vi "输入输出力计算.vi"(6 "测量点数组":dbl[](array[numeric]), 7 "滞后监控点":dbl, 8 "左下降数组":dbl[][](array[numeric]), 9 "左上升数组":dbl[][](array[numeric]), 10 "右下降数组":dbl[][](array[numeric]), 11 "右上升数组":dbl[][](array[numeric])) -> (1 "扭差":dbl, 2 "左扭矩数组":dbl[](array[numeric]), 3 "右扭矩数组":dbl[](array[numeric]), 4 "左滞后":dbl, 5 "右滞后":dbl)   [LabVIEW 2011]
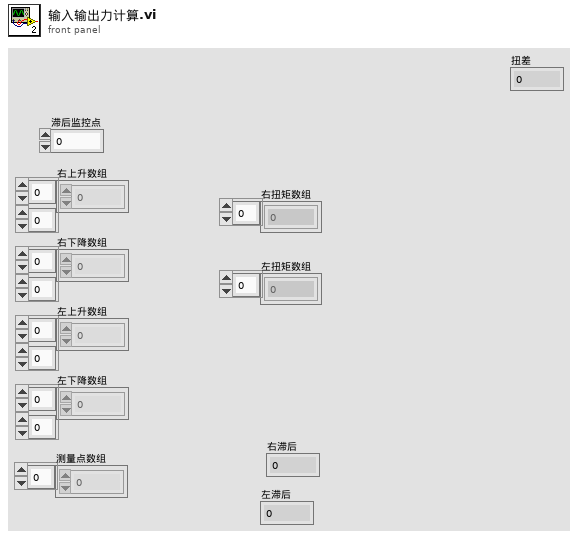
[diagram p1: front panel]
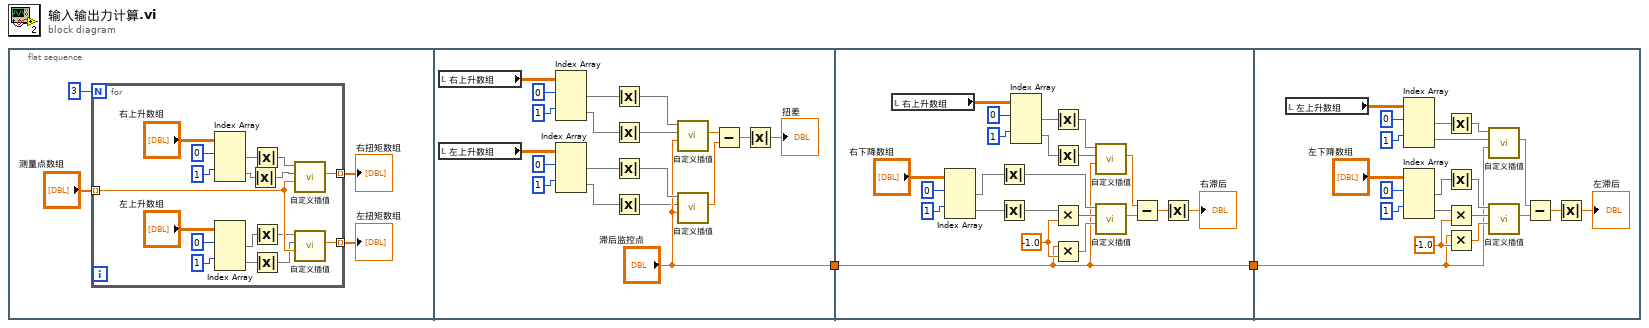
[diagram p0: block diagram]
diagram:
  n1 = flat-sequence {
    tunnel: ["滞后监控点"] -> w1
    tunnel: [w47] -> w2
    tunnel: w1 -> [w47]
    tunnel: w2 -> [w67]
    frame #0 {
      n2 = for {
        N: 3 -> [_]
        tunnel: "测量点数组" -> [w19] mode=indexing
        tunnel: [w14] -> w4 mode=indexing
        tunnel: [w13] -> w3 mode=indexing
        n3 = Index Array(array="右上升数组", index (row) #1=0 ("索引 (行)"), index (row) #2=1 ("索引 (行)")) -> (element #1=w18:dbl[], element #2=w8:dbl[])  [unwired: 2 in]
        n4 = Index Array(array="左上升数组", index (row) #1=0 ("索引 (行)"), index (row) #2=1 ("索引 (行)")) -> (element #1=w16:dbl[], element #2=w10:dbl[])  [unwired: 2 in]
        n5 = Absolute Value(x=w8) -> (abs(x)=w7:dbl[])
        n6 = Absolute Value(x=w18) -> (abs(x)=w17:dbl[])
        n7 = Absolute Value(x=w16) -> (abs(x)=w15:dbl[])
        n8 = Absolute Value(x=w10) -> (abs(x)=w9:dbl[])
        n9 = call "自定义插值.vi"("压力"=w19, "压力数组"=w7, "扭矩数组"=w17) -> ("扭矩值"=w14:dbl)  [unwired: 8 in]
        n10 = call "自定义插值.vi"("压力"=w19, "压力数组"=w9, "扭矩数组"=w15) -> ("扭矩值"=w13:dbl)  [unwired: 8 in]
      }
      "右扭矩数组" <- w4
      "左扭矩数组" <- w3
    }
    frame #1 {
      n11 = local read "右上升数组"() -> (w40:dbl[][])
      n12 = local read "左上升数组"() -> (w37:dbl[][])
      n13 = Index Array(array=w40, index (row) #1=0 ("索引 (行)"), index (row) #2=1 ("索引 (行)")) -> (element #1=w36:dbl[], element #2=w25:dbl[])  [unwired: 2 in]
      n14 = Index Array(array=w37, index (row) #1=0 ("索引 (行)"), index (row) #2=1 ("索引 (行)")) -> (element #1=w33:dbl[], element #2=w27:dbl[])  [unwired: 2 in]
      n15 = Absolute Value(x=w36) -> (abs(x)=w35:dbl[])
      n16 = Absolute Value(x=w25) -> (abs(x)=w24:dbl[])
      n17 = Absolute Value(x=w33) -> (abs(x)=w34:dbl[])
      n18 = Absolute Value(x=w27) -> (abs(x)=w26:dbl[])
      n19 = call "自定义插值.vi"("压力"="滞后监控点", "压力数组"=w24, "扭矩数组"=w35) -> ("扭矩值"=w32:dbl)  [unwired: 8 in]
      n20 = call "自定义插值.vi"("压力"="滞后监控点", "压力数组"=w26, "扭矩数组"=w34) -> ("扭矩值"=w31:dbl)  [unwired: 8 in]
      n21 = Subtract(x=w32, y=w31) -> (x-y=w29:dbl)
      n22 = Absolute Value(x=w29) -> (abs(x)=→"扭差":dbl)
    }
    frame #2 {
      w52 = -1.0 ("y")
      n23 = local read "右上升数组"() -> (w60:dbl[][])
      n24 = Index Array(array="右下降数组", index (row) #1=0 ("索引 (行)"), index (row) #2=1 ("索引 (行)")) -> (element #1=w58:dbl[], element #2=w44:dbl[])  [unwired: 2 in]
      n25 = Absolute Value(x=w58) -> (abs(x)=w57:dbl[])
      n26 = Absolute Value(x=w44) -> (abs(x)=w43:dbl[])
      n27 = Index Array(array=w60, index (row) #1=0 ("索引 (行)"), index (row) #2=1 ("索引 (行)")) -> (element #1=w63:dbl[], element #2=w46:dbl[])  [unwired: 2 in]
      n28 = Absolute Value(x=w63) -> (abs(x)=w62:dbl[])
      n29 = Absolute Value(x=w46) -> (abs(x)=w45:dbl[])
      n30 = Multiply(x=w43, y=w52) -> (x*y=w54:dbl[])
      n31 = Multiply(x=w47, y=w52) -> (x*y=w53:dbl)
      n32 = call "自定义插值.vi"("压力"=w47, "压力数组"=w45, "扭矩数组"=w62) -> ("扭矩值"=w50:dbl)  [unwired: 8 in]
      n33 = call "自定义插值.vi"("压力"=w53, "压力数组"=w54, "扭矩数组"=w57) -> ("扭矩值"=w49:dbl)  [unwired: 8 in]
      n34 = Subtract(x=w50, y=w49) -> (x-y=w51:dbl)
      n35 = Absolute Value(x=w51) -> (abs(x)=→"右滞后":dbl)
    }
    frame #3 {
      w72 = -1.0 ("y")
      n36 = local read "左上升数组"() -> (w65:dbl[][])
      n37 = Index Array(array=w65, index (row) #1=0 ("索引 (行)"), index (row) #2=1 ("索引 (行)")) -> (element #1=w82:dbl[], element #2=w83:dbl[])  [unwired: 2 in]
      n38 = Index Array(array="左下降数组", index (row) #1=0 ("索引 (行)"), index (row) #2=1 ("索引 (行)")) -> (element #1=w78:dbl[], element #2=w75:dbl[])  [unwired: 2 in]
      n39 = Absolute Value(x=w82) -> (abs(x)=w81:dbl[])
      n40 = Absolute Value(x=w78) -> (abs(x)=w77:dbl[])
      n41 = Multiply(x=w75, y=w72) -> (x*y=w74:dbl[])
      n42 = Multiply(x=w67, y=w72) -> (x*y=w73:dbl)
      n43 = call "自定义插值.vi"("压力"=w67, "压力数组"=w83, "扭矩数组"=w81) -> ("扭矩值"=w70:dbl)  [unwired: 8 in]
      n44 = call "自定义插值.vi"("压力"=w73, "压力数组"=w74, "扭矩数组"=w77) -> ("扭矩值"=w69:dbl)  [unwired: 8 in]
      n45 = Subtract(x=w70, y=w69) -> (x-y=w71:dbl)
      n46 = Absolute Value(x=w71) -> (abs(x)=→"左滞后":dbl)
    }
  }
